vi "Read Channel Info.vi"(8 "error in (no error)":errorcluster, 11 "Lockin SR830.lvclass in":refnum<class "Lockin SR830.lvclass">) -> (0 "error out":errorcluster, 1 "Channel Units":string[](array[string]), 2 "Channel Names":string[](array[string]), 3 "Lockin SR830.lvclass out":refnum<class "Lockin SR830.lvclass">, 5 "#Channels":i32)   [LabVIEW 2009, in "Lockin SR830.lvclass"]
doc: "(Dynamic) Return information about the readable data channels this object provides, e.g., the name of each data source and its unit."
uses:
  Lockin SR830.lvclass
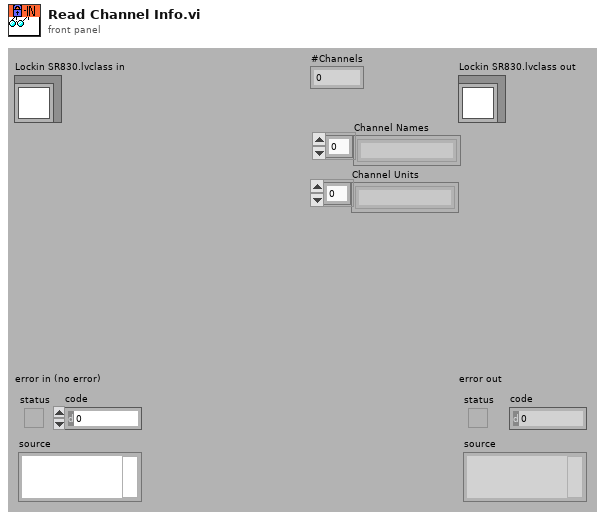
[diagram p1: front panel]
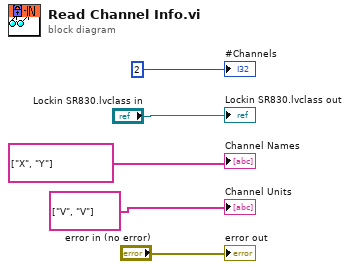
[diagram p0: block diagram]
diagram:
  "error out" <- "error in (no error)"
  "Lockin SR830.lvclass out" <- "Lockin SR830.lvclass in"
  "Channel Units" <- string[] ["V", "V"] ("Channel Units")
  "Channel Names" <- string[] ["X", "Y"] ("Channel Names")
  "#Channels" <- 2 ("#Channels")
